vi "Periodic Tasks.vi"(8 "error in":errorcluster) -> ()   [LabVIEW 2018]
doc: "This VI runs in parallel to other tasks. It can contain as many user-defined periodic loops as you need. These can carry out PID or other sorts of timed response."
uses:
  <vilib>/Analysis/coordinate.llb/Angle Range (Degree).ctl
  <vilib>/Analysis/coordinate.llb/Angle Units.ctl
  <vilib>/Analysis/coordinate.llb/Wrap Angle (scalar).vi
  <vilib>/Rock Robotics/WPI/Utilities/WPI_GetSetVariantRefNum.vi
  MyGlobal.vi
  <vilib>/Analysis/NI_AAL_Angle.lvlib
panel:
  out "Distance":dbl
  out "result":bool
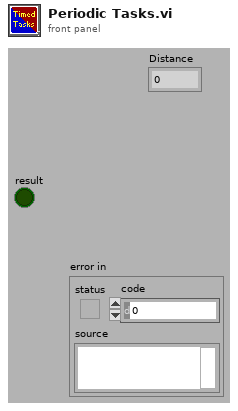
[diagram p1: front panel]
types:
  T1 = typedef "WPI_JoystickDevRef.ctl" = cluster{"Device":T2}
  T2 = typedef "WPI_JoystickDeviceEnum.ctl" = enum16{"USB 0", "USB 1", "USB 2", "USB 3", "USB 4", "USB 5"}
  T3 = typedef "WPI_RobotDriveDevRef.ctl" = cluster{"DevStatus":errorcluster, "Motors[]":T4[], "Square Inputs":bool, "Max Output":dbl}
  T4 = typedef "WPI_MotorControlDeviceRef.ctl" = cluster{"DeviceStatus":errorcluster, "Type":T5, "PWM":cluster{"PWM Channel":T6, "DeadBand":T7}, "CAN":cluster{"Device Number":u8, "SetOutput VI Ref":variant, "GetOutput VI Ref":variant, "Enable VI Ref":variant, "Disable VI Ref":variant, "Data":variant}, "Invert":bool, "DIO PWM":cluster{"PWM \"Enable\" Channel":T6, "DIOChannel":T8, "PWM Rate":dbl}}
  T5 = typedef "WPI_MotorControlType.ctl" = enum16{"PWM", "CAN", "DIO PWM"}
  T6 = typedef "FPGA_DIOPWMChannel.ctl" = enum8{"PWM 0", "PWM 1", "PWM 2", "PWM 3", "PWM 4", "PWM 5", "PWM 6", "PWM 7", "PWM 8", "PWM 9", "PWM MXP 0", "PWM MXP 1", "PWM MXP 2", "PWM MXP 3", "PWM MXP 4", "PWM MXP 5", "PWM MXP 6", "PWM MXP 7", "PWM MXP 8", "PWM MXP 9", "Invalid"}
  T7 = typedef "WPI_PWMDeadband.ctl" = cluster{"Name":string, "maxPositivePwm":i32, "minPositivePwm":i32, "centerPwm":i32, "maxNegativePwm":i32, "minNegativePwm":i32, "angularRange":u16}
  T8 = typedef "FPGA_DIOChannel.ctl" = enum8{"DIO 0", "DIO 1", "DIO 2", "DIO 3", "DIO 4", "DIO 5", "DIO 6", "DIO 7", "DIO 8", "DIO 9", "DIO MXP 0", "DIO MXP 1", "DIO MXP 2", "DIO MXP 3", "DIO MXP 4", "DIO MXP 5", "DIO MXP 6", "DIO MXP 7", "DIO MXP 8", "DIO MXP 9", "DIO MXP 10", "DIO MXP 11", "DIO MXP 12", "DIO MXP 13", "DIO MXP 14", "DIO MXP 15", "SPI Port CS1", "SPI Port CS2", "SPI Port CS3", "SPI Port MISO", "SPI Port MOSI", "Invalid"}
  T9 = cluster{"JoystickDevRef":T1, "RobotDriveDevRef":T3}
  T10 = typedef "Drivetype.ctl" = enum16{"4 vitesse", "1 vitesse"}
  T11 = typedef "SwerveDrive.ctl" = cluster{"AVD":cluster{"Angle":dbl, "Vitesse":dbl}, "AVG":cluster{"Angle":dbl, "Vitesse":dbl}, "ARG":cluster{"Angle":dbl, "Vitesse":dbl}, "ARD":cluster{"Angle":dbl, "Vitesse":dbl}}
  T12 = typedef "NI_AAL_Angle.lvlib/Angle Units.ctl" = i32
  T13 = typedef "NI_AAL_Angle.lvlib/Angle Range (Degree).ctl" = u16
  T14 = typedef "WPI_I2CDevRef.ctl" = cluster{"DevStatus":errorcluster, "Device Address":u8, "Handle":i32, "I2C Bus":T15}
  T15 = typedef "i2c_bus.ctl" = enum16{"I2C On-Board", "I2C MXP", "Invalid"}
  T16 = typedef "WPI_AnalogChannelDevRef.ctl" = cluster{"DevStatus":errorcluster, "Analog Channel":T17}
  T17 = typedef "FPGA_AIChannel.ctl" = enum8{"AI 0", "AI 1", "AI 2", "AI 3", "AI MXP 0", "AI MXP 1", "AI MXP 2", "AI MXP 3", "Invalid"}
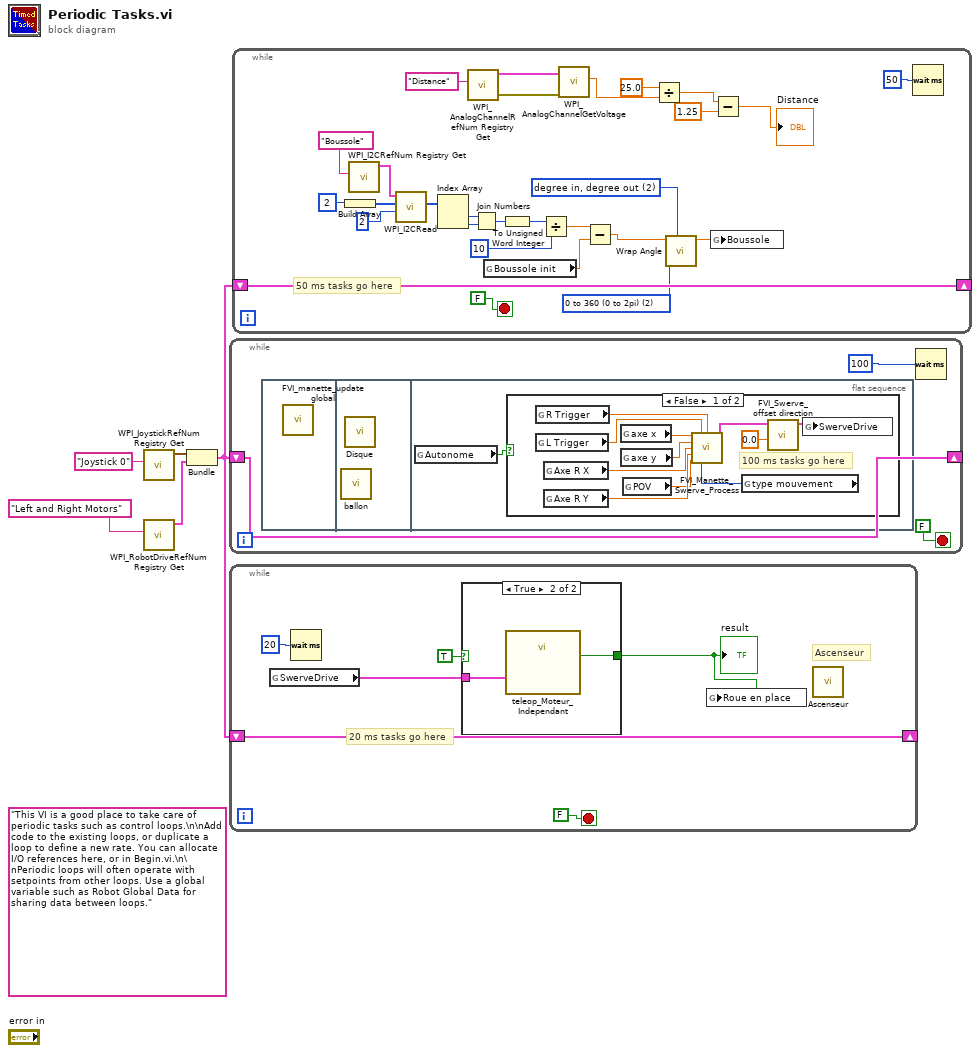
[diagram p0: block diagram]
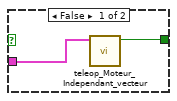
[diagram p2: hidden frame]
diagram:
  (unwired) "This VI is a good place to take care of periodic tasks such as control loops.\n\nAdd code to the existing loops, or duplicate a loop to define a new rate. You can allocate I/O references here, or in Begin.vi.\n\nPeriodic loops will often operate with setpoints from other loops. Use a global variable such as Robot Global Data for sharing data between loops."
  n1 = call <vilib>:"WPI_JoystickRefNum Registry Get.vi"("refnum name"="Joystick 0") -> ("JoystickDevRef"=w3:T1)  [unwired: 1 in, 9 out]
  n2 = call <vilib>:"WPI_RobotDriveRefNum Registry Get.vi"("refnum name"="Left and Right Motors") -> ("RobotDriveDevRef"=w2:T3)  [unwired: 1 in, 9 out]
  n3 = Bundle("JoystickDevRef"=w3, "RobotDriveDevRef"=w2) -> (w1:T9)  [unwired: 1 out]
  n4 = while {
    shift-right: [w7] -> _
    shift-left: w1 -> [w7]
    stop <- FALSE stop-if-true
    n5 = flat-sequence {
      frame #0 {
        n6 = call "FVI_manette_update global.vi"() -> ()  [unwired: 12 in]
      }
      frame #1 {
        n7 = call "ballon.vi"() -> ()  [unwired: 12 in]
        n8 = call "Disque.vi"() -> ()  [unwired: 12 in]
      }
      frame #2 {
        n9 = global read "MyGlobal.vi" "Autonome"() -> (w9:bool)
        n10 = case shown="False" w9 {
          frame False {
            # "100 ms tasks go here"
            n11 = global read "MyGlobal.vi" "R Trigger"() -> (w15:dbl)
            n12 = global read "MyGlobal.vi" "L Trigger"() -> (w16:dbl)
            n13 = global read "MyGlobal.vi" "Axe R X"() -> (w20:dbl)
            n14 = global read "MyGlobal.vi" "Axe R Y"() -> (w19:dbl)
            n15 = global read "MyGlobal.vi" "axe x"() -> (w18:dbl)
            n16 = global read "MyGlobal.vi" "axe y"() -> (w17:dbl)
            n17 = global read "MyGlobal.vi" "POV"() -> (w14:dbl)
            n18 = global read "MyGlobal.vi" "type mouvement"() -> (w13:T10)
            n19 = call "FVI_Manette_Swerve_Process.vi"("Axe L X"=w18, "Ltrigger"=w16, "Rtrigger"=w15, "Axe L Y"=w17, "Axe R X"=w20, "Axe R Y"=w19, "POV"=w14, "type mouvement"=w13) -> ("SwerveDrive"=w12:T11)  [unwired: 7 in]
            n20 = call "FVI_Swerve_offset direction.vi"("Correction angle"=0.0, "SwerveDrive in"=w12) -> ("SwerveDrive out"=w11:T11)  [unwired: 9 in]
            n21 = global write "MyGlobal.vi" "SwerveDrive"(w11) -> ()
          }
          frame True {
          }
        }
      }
    }
    n22 = Wait (ms)(milliseconds to wait=u32 100) -> ()  [unwired: 1 out]
  }
  n23 = while {
    shift-right: [w24] -> _
    shift-left: w1 -> [w24]
    stop <- FALSE stop-if-true
    # "Ascenseur"
    # "20 ms tasks go here"
    n24 = global read "MyGlobal.vi" "SwerveDrive"() -> (w23:T11)
    n25 = Wait (ms)(milliseconds to wait=u32 20) -> ()  [unwired: 1 out]
    n26 = case shown="True" TRUE {
      tunnel: w23 -> [w28 w30]
      tunnel: [w27 w29] -> w22
      frame False {
        n27 = call "teleop_Moteur_Independant_vecteur.vi"("SwerveDrive"=w28) -> ("result"=w27:bool)  [unwired: 10 in]
      }
      frame True {
        n28 = call "teleop_Moteur_Independant.vi"("SwerveDrive"=w30) -> ("result"=w29:bool)  [unwired: 10 in]
      }
    }
    "result" <- w22
    n29 = global write "MyGlobal.vi" "Roue en place"(w22) -> ()
    n30 = call "Ascenseur.vi"() -> ()  [unwired: 12 in]
  }
  n31 = while {
    shift-right: [w56] -> _
    shift-left: w1 -> [w56]
    stop <- FALSE stop-if-true
    w40 = T12 2 items=["radian in, radian out", "radian in, degree out", "degree in, degree out", "degree in, radian out"] ("angle units")
    w42 = T13 2 items=["none", "-180 to 180 (-pi to pi)", "0 to 360 (0 to 2pi)"] ("angle range")
    # "50 ms tasks go here"
    n32 = Build Array(u8 2 ("Data To Send")) -> (w53:u8[])
    n33 = call <vilib>:"WPI_I2CRefNum Registry Get.vi"("refnum name"="Boussole") -> ("I2CDevRef"=w46:T14)  [unwired: 9 in, 1 out]
    n34 = call <vilib>:"WPI_I2CRead.vi"("I2CBytesToRead"=u8 2, "I2CRegister"=w53, "I2CDevRef"=w46) -> ("Data Out"=w55:u8[])  [unwired: 1 in, 7 out]
    n35 = Index Array(array=w55) -> (element #1=w50:u8, element #2=w49:u8)  [unwired: 2 in]
    n36 = call <vilib>:"WPI_AnalogChannelRefNum Registry Get.vi"("refnum name"="Distance") -> ("error out"=w37:errorcluster, "AIDeviceRef"=w38:T16)  [unwired: 9 in]
    n37 = Join Numbers(hi=w50, lo=w49) -> ((hi.lo)=w54:u16)
    n38 = global read "MyGlobal.vi" "Boussole init"() -> (w44:dbl)
    n39 = To Unsigned Word Integer(number=w54) -> (unsigned 16bit integer=w48:u16)
    n40 = Divide(x=w48, y=u16 10) -> (x/y=w45:dbl)
    n41 = call <vilib>:"WPI_AnalogChannelGetVoltage.vi"("error in (no error)"=w37, "AIDeviceRef"=w38) -> ("Voltage"=w35:dbl)  [unwired: 7 in, 2 out]
    n42 = Subtract(x=w45, y=w44) -> (x-y=w43:dbl)
    n43 = Divide(x=25.0, y=w35) -> (x/y=w32:dbl)
    n44 = call-poly <vilib>:"Wrap Angle.vi"("angle units"=w40, "angle range"=w42, "angle in"=w43) -> ("angle out"=w41:dbl)  [unwired: 7 in, 1 out]
    n45 = global write "MyGlobal.vi" "Boussole"(w41) -> ()
    n46 = Subtract(x=w32, y=1.25) -> (x-y=→"Distance":dbl)
    n47 = Wait (ms)(milliseconds to wait=u32 50) -> ()  [unwired: 1 out]
  }
